vi "Get Refnum From Indexing Terminal.vi"(8 "error in":errorcluster, 11 "Refnum Terminal":refnum<vi>) -> (0 "error out":errorcluster, 1 "Indexing term found?":bool, 2 "Chosen Terminal":refnum<vi>, 3 "Terminal Data Cluster":T1)   [LabVIEW 2023]
doc: "Determine if terminal is on an indexing tunnel, and report which side of the tunnel is the refnum side (choice 1 = ouside structure, chce 2 = inside structure)\n\nThis VI returns the refnum terminal side of an indexing terminal (or the input value if it was already a refnum terminal)."
panel:
  # "non-array terminal is input is indexing"
  # "can be refnum or cluster type"
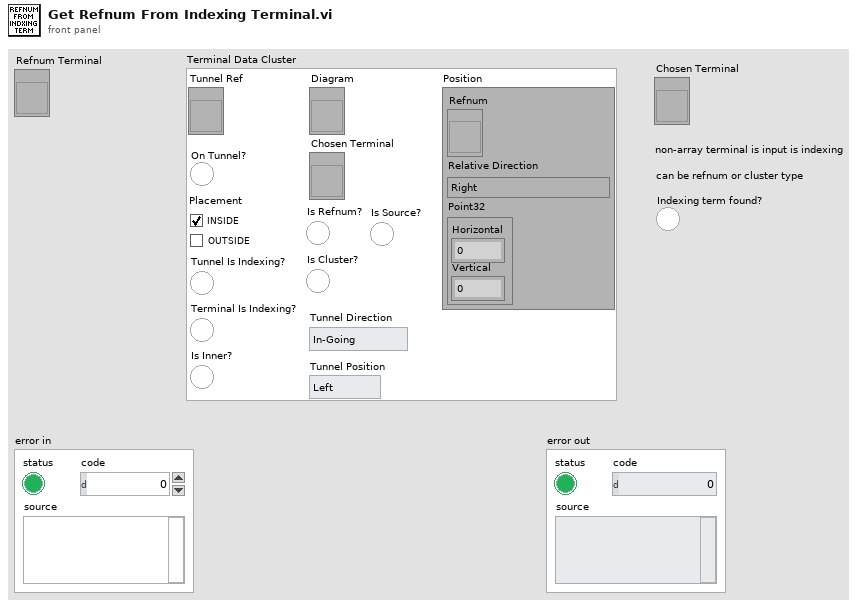
[diagram p1: front panel]
types:
  T1 = cluster{"Tunnel Ref":refnum<vi>, "On Tunnel?":bool, "Placement":enum32{"Choice 1", "Choice 2"}, "Tunnel Is Indexing?":bool, "Diagram":refnum<vi>, "Position":cluster{"Refnum":refnum<vi>, "Relative Direction":enum32{"Right", "Left", "Top", "Bottom", "Top Right", "Top Left", "Bottom Right", "Bottom Left"}, "Point32":cluster{"Horizontal":i32, "Vertical":i32}}, "Chosen Terminal":refnum<vi>, "Is Refnum?":bool, "Is Cluster?":bool, "Is Source?":bool, "Tunnel Direction":enum16{"In-Going", "Out-Going"}, "Tunnel Position":enum16{"Left", "Top", "Right", "Bottom"}, "Is Inner?":bool, "Terminal Is Indexing?":bool}
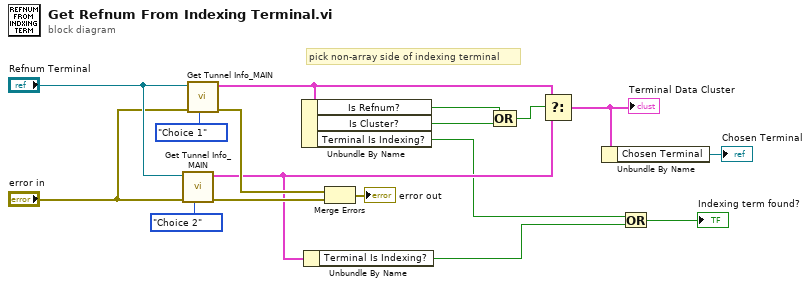
[diagram p0: block diagram]
diagram:
  # "pick non-array side of indexing terminal"
  n1 = call "Get Tunnel Info_MAIN.vi"("Object Placement"=enum32{"Choice 1", "Choice 2"}."Choice 2", "error in"="error in", "Terminal in"="Refnum Terminal") -> ("error out"=w14:errorcluster, "Terminal Data Cluster"=w3:T1)  [unwired: 6 in, 1 out]
  n2 = call "Get Tunnel Info_MAIN.vi"("Object Placement"=enum32{"Choice 1", "Choice 2"}."Choice 1", "error in"="error in", "Terminal in"="Refnum Terminal") -> ("error out"=w13:errorcluster, "Terminal Data Cluster"=w15:T1)  [unwired: 6 in, 1 out]
  n3 = Unbundle By Name(w15) -> ("Is Refnum?"=w8:bool, "Is Cluster?"=w9:bool, "Terminal Is Indexing?"=w2:bool)
  n4 = Unbundle By Name(w3) -> ("Terminal Is Indexing?"=w1:bool)
  n5 = Merge Errors(w13, w14) -> (→"error out":errorcluster)
  n6 = Compound Arithmetic op=OR(w8, w9) -> (w7:bool)
  n7 = Select(t=w15, s=w7, f=w3) -> (s? t:f=w6:T1)
  "Terminal Data Cluster" <- w6
  n8 = Unbundle By Name(w6) -> ("Chosen Terminal"=→"Chosen Terminal":refnum<vi>)
  n9 = Or(x=w2, y=w1) -> (x .or. y?=→"Indexing term found?":bool)
